vi "State Machine 1.vi"   [LabVIEW 2022 SP3]
panel:
  # "State"
  # "Start\n\nProcess 1\n\nProcess 2\n\nStop"
  # "start"
  # "Process 1"
  # "Process 2"
  # "Stop"
types:
  T1 = enum16{"Start", "Process 1", "Process 2", "Stop"}
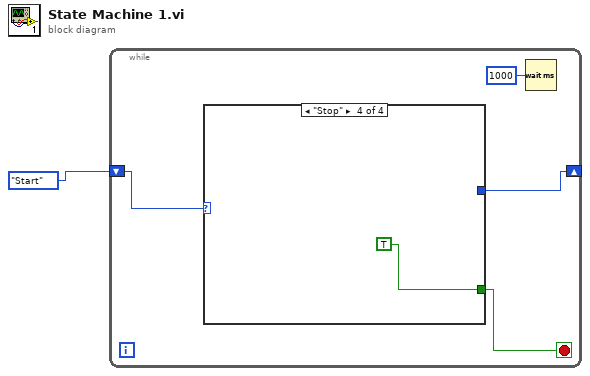
[diagram p0: block diagram]
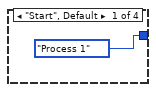
[diagram p2: hidden frame]
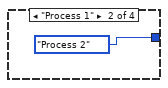
[diagram p3: hidden frame]
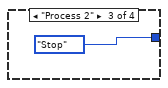
[diagram p4: hidden frame]
diagram:
  n1 = while {
    shift-right: [w3] -> _
    shift-left: T1."Start" -> [w5]
    stop <- w2 stop-if-true
    n2 = case shown="\"Stop\"" w5 {
      tunnel: [T1."Process 1" T1."Process 2" T1."Stop" _] -> w3
      tunnel: [_ _ _ TRUE] -> w2
      frame "Start", Default {
      }
      frame "Process 1" {
      }
      frame "Process 2" {
      }
      frame "Stop" {
      }
    }
    n3 = Wait (ms)(milliseconds to wait=u32 1000) -> ()  [unwired: 1 out]
  }
